vi "Get Output DMA Refs.vi"(8 "error in (no error)":errorcluster, 10 "Item GUID":string, 11 "Section Ref in":T1 format="%.0x") -> (0 "error out":errorcluster, 1 "Refs":T2(array[cluster]) {"VS Refs" format="%.0x"}, 2 "DMA":T3[](array[typedef]) {"Data Type" format="%.0x"; "DMA.Settings"."DMA Host Buffer" items=["1 Second"=1, "2 Seconds"=2, "5 Seconds"=5, "10 Seconds"=10]; "DMA.Settings"."dt" format="%#_p"; "DMA.Settings"."Update Rate" items=["1 Hz"=1, "2 Hz"=2, "5 Hz"=5, "10 Hz"=10]}, 3 "Section Ref out":T1 format="%.0x")   [LabVIEW 2020, in "FPGA Addon System Explorer.lvlib"]
uses:
  FPGA Addon System Explorer.lvlib
  <vilib>/NI VeriStand/Custom Device API/Custom Device Item Ref.ctl
  Addon Shared/Types/Compiled.DMASettings.ctl
  Addon Shared/Types/FPGA Addon Data Type.ctl
  Addon Shared/Types/DMA Settings.ctl
  Addon Shared/Types/Delacing Scheme.ctl
  Addon Shared/Types/DMA Acquisition Mode.ctl
  <vilib>/NI VeriStand/Custom Device API/Waveform Data Reference.ctl
  Addon Shared/Types/FG Action.ctl
  Addon Shared/SubVIs/Constants.vi
  <vilib>/NI VeriStand/Custom Device Tools/Custom Device Utility Library/NI VeriStand - Search for Item by GUID.vi
  <vilib>/NI/NI VeriStand Advanced SysDef API/SysDef API/SysDef.Property.Get.vi
  <vilib>/NI/NI VeriStand Advanced SysDef API/_SubVIs/SysDef.Property.Get.Variant.vi
  <vilib>/NI/NI VeriStand Advanced SysDef API/SysDef API/SysDef.Property.Set.vi
  <vilib>/NI/NI VeriStand Advanced SysDef API/_SubVIs/SysDef.Property.Set.Variant.vi
  <vilib>/NI VeriStand/Custom Device API/Get Item Property (String).vi
  <vilib>/NI VeriStand/Custom Device API/Get Item Property (U32).vi
  <vilib>/NI VeriStand/Custom Device API/Get Item Property (Double).vi
  <vilib>/NI VeriStand/Custom Device API/NI VeriStand - Set Item Property.vi
  <vilib>/NI VeriStand/Custom Device API/Set Item Property (U32).vi
  <vilib>/NI VeriStand/Custom Device API/Set Item Property (Double).vi
  <vilib>/NI VeriStand/Custom Device Tools/Custom Device Utility Library/NI VeriStand - Search for All Items by GUID.vi
  <vilib>/NI VeriStand/Custom Device API/Get Item Property (Dependent Node Pointer).vi
  Addon Shared/FPGA Addon Shared.lvlib
  <vilib>/NI VeriStand/Custom Device API/Custom Device API.lvlib
  <vilib>/NI VeriStand/Custom Device Tools/Custom Device Utility Library/Custom Device Utility Library.lvlib
  <vilib>/NI VeriStand/Custom Device Tools/Custom Device Utility Library/NI VeriStand - Search for Item by Name.vi
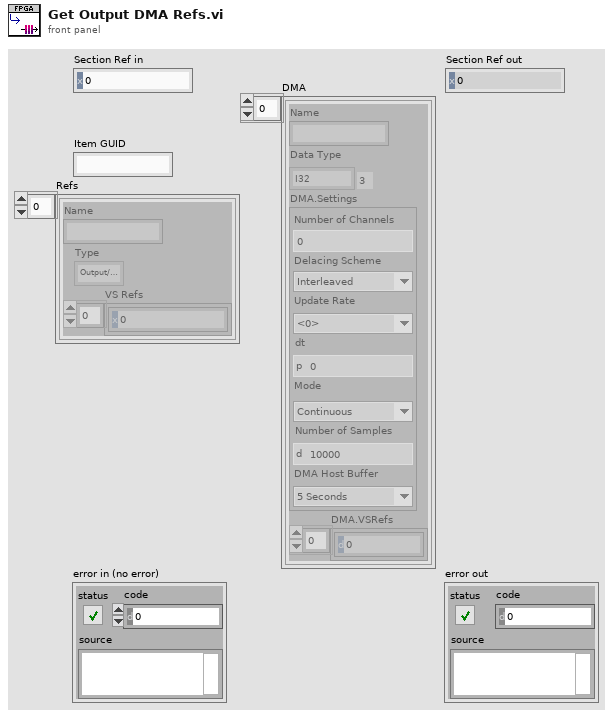
[diagram p1: front panel]
types:
  T1 = typedef "Custom Device API.lvlib/Custom Device Item Ref.ctl" = u64
  T2 = cluster{"Name":string, "Type":enum16{"Output/Write", "Input/Read", "Input/ReadWrite"}, "VS Refs":T1[]}[]
  T3 = typedef "FPGA Addon Shared.lvlib/Compiled.DMASettings.ctl" = cluster{"Name":string, "Data Type":T4, "DMA.Settings":T5, "DMA.VSRefs":T8[]}
  T4 = typedef "FPGA Addon Shared.lvlib/FPGA Addon Data Type.ctl" = enum8{"<Null>", "I8", "I16", "I32", "I64", "U8", "U16", "U32", "U64", "SGL", "Boolean", "Analog PWM In Settings", "Analog PWM In", "Digital PWM In Settings", "Digital PWM In", "Digital PWM Out", "Sine Out", "FXP", "FXP+/-24.5", "FXP+/-16.5", "FXP+/-32.8", "FXP+/-64.32", "FXP+/-16.7", "FXP+/-20.5", "FXP+/-27.5", "FXP+/-32.16", "FXP+16.3", "FXP+18.3", "Digital Static In", "Digital Static Out", "Digital Static In Settings", "Digital WSS Out", "Quad Encoder Settings", "Quad Encoder In", "Group"}
  T5 = typedef "FPGA Addon Shared.lvlib/DMA Settings.ctl" = cluster{"Number of Channels":u8, "Delacing Scheme":T6, "Update Rate":u32, "dt":dbl, "Mode":T7, "Number of Samples":u32, "DMA Host Buffer":u32}
  T6 = typedef "FPGA Addon Shared.lvlib/Delacing Scheme.ctl" = enum8{"Interleaved", "Bitpacked"}
  T7 = typedef "FPGA Addon Shared.lvlib/DMA Acquisition Mode.ctl" = enum8{"Continuous", "Triggered Finite"}
  T8 = typedef "Custom Device API.lvlib/Waveform Data Reference.ctl" = i32
  T9 = typedef "FPGA Addon Shared.lvlib/FG Action.ctl" = enum8{"GET", "SET"}
  T10 = typedef "FPGA Addon Shared.lvlib/DMA Information.ctl" = cluster{"Name":string, "Data Type":T4}
  T11 = cluster{"Name":string, "Type":enum16{"Output/Write", "Input/Read", "Input/ReadWrite"}, "VS Refs":T1[]}
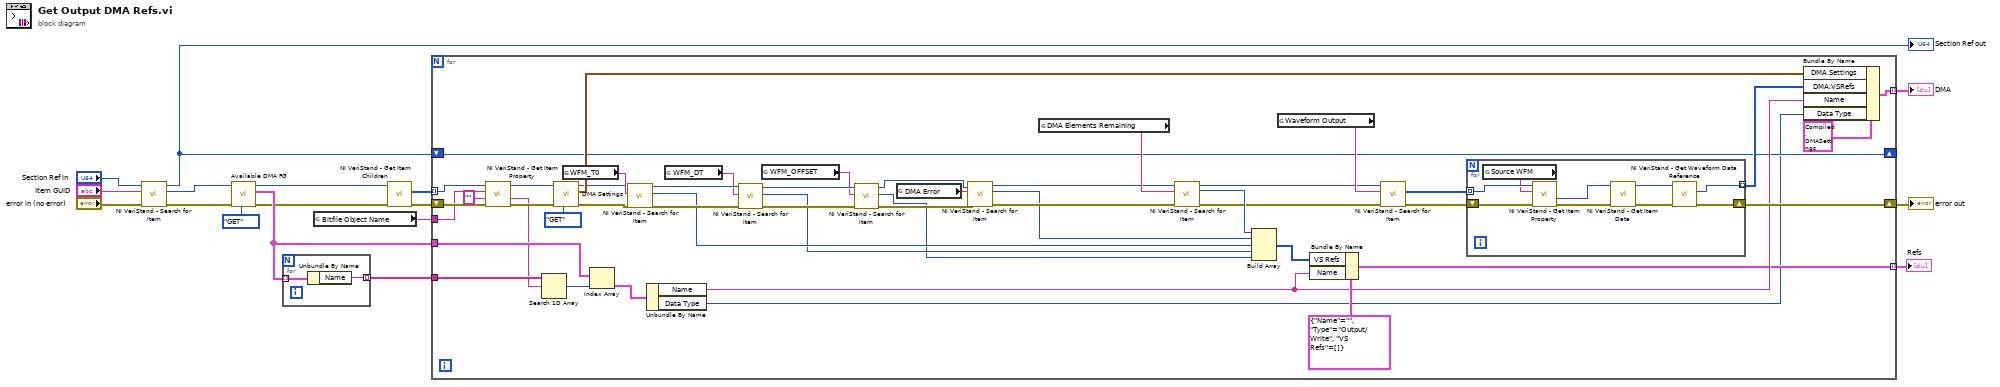
[diagram p0: block diagram]
diagram:
  n1 = call-poly <vilib>:"NI VeriStand - Search for Item.vi"("error in"="error in (no error)", "Item GUID"="Item GUID", "Section Ref in"="Section Ref in") -> ("error out"=w14:errorcluster, "Item Ref"=w16:T1, "Section Ref out"=w3:T1)  [unwired: 5 in, 1 out]
  "Section Ref out" <- w3
  n2 = call "Available DMA FG.vi"("Action"=FG_Action."GET", "error in (no error)"=w14, "Item Ref"=w16) -> ("error out"=w10:errorcluster, "Available DMA"=w11:T10[], "Item Ref out"=w12:T1)  [unwired: 6 in]
  n3 = for {
    tunnel: w11 -> [w19] mode=indexing
    tunnel: [w18] -> w9 mode=indexing
    n4 = Unbundle By Name(w19) -> ("Name"=w18:string)
  }
  n5 = global read "Constants.vi" "Bitfile Object Name"() -> (w8:string)
  n6 = call <vilib>:"NI VeriStand - Get Item Children.vi"("error in (no error)"=w10, "Item Ref in"=w12) -> ("error out"=w6:errorcluster, "Child Refs"=w7:T1[])  [unwired: 6 in, 2 out]
  n7 = for {
    shift-right: [w42] -> w4
    shift-left: w6 -> [w67]
    tunnel: w7 -> [w66] mode=indexing
    tunnel: w8 -> [w65]
    tunnel: w9 -> [w63]
    tunnel: w11 -> [w62]
    tunnel: [w57] -> w2 mode=indexing
    shift-right: [w35] -> _
    shift-left: w3 -> [w35]
    tunnel: [w37] -> w1 mode=indexing
    n8 = call-poly <vilib>:"NI VeriStand - Get Item Property.vi"("error in (no error)"=w67, "Default Value"="", "Property Name"=w65, "Item Ref in"=w66) -> ("error out"=w56:errorcluster, "Value"=w52:string, "Item Ref out"=w55:T1)  [unwired: 4 in, 1 out]
    n9 = Search 1D Array(1D array=w63, element=w52) -> (index of element=w61:i32)  [unwired: 1 in]
    n10 = call "DMA Settings.vi"("Action"=FG_Action."GET", "error in (no error)"=w56, "Item Ref"=w55) -> ("error out"=w23:errorcluster, "DMA Settings"=w44:T5, "Item Ref out"=w24:T1)  [unwired: 6 in]
    n11 = global read "Constants.vi" "WFM_T0"() -> (w29:string)
    n12 = Index Array(array=w62, index=w61) -> (element=w59:T10)
    n13 = call-poly <vilib>:"NI VeriStand - Search for Item.vi"("error in"=w23, "Item Name"=w29, "Section Ref in"=w24) -> ("error out"=w32:errorcluster, "Item Ref"=w22:T1, "Section Ref out"=w33:T1)  [unwired: 5 in, 1 out]
    n14 = Unbundle By Name(w59) -> ("Name"=w38:string, "Data Type"=w34:T4)
    n15 = global read "Constants.vi" "WFM_DT"() -> (w28:string)
    n16 = call-poly <vilib>:"NI VeriStand - Search for Item.vi"("error in"=w32, "Item Name"=w28, "Section Ref in"=w33) -> ("error out"=w30:errorcluster, "Item Ref"=w21:T1, "Section Ref out"=w31:T1)  [unwired: 5 in, 1 out]
    n17 = global read "Constants.vi" "WFM_OFFSET"() -> (w27:string)
    n18 = call-poly <vilib>:"NI VeriStand - Search for Item.vi"("error in"=w30, "Item Name"=w27, "Section Ref in"=w31) -> ("error out"=w25:errorcluster, "Item Ref"=w20:T1, "Section Ref out"=w26:T1)  [unwired: 5 in, 1 out]
    n19 = global read "Constants.vi" "DMA Error"() -> (w51:string)
    n20 = call-poly <vilib>:"NI VeriStand - Search for Item.vi"("error in"=w25, "Item GUID"=w51, "Section Ref in"=w26) -> ("error out"=w49:errorcluster, "Item Ref"=w47:T1, "Section Ref out"=w48:T1)  [unwired: 5 in, 1 out]
    n21 = global read "Constants.vi" "DMA Elements Remaining"() -> (w50:string)
    n22 = call-poly <vilib>:"NI VeriStand - Search for Item.vi"("error in"=w49, "Item GUID"=w50, "Section Ref in"=w48) -> ("error out"=w36:errorcluster, "Item Ref"=w46:T1, "Section Ref out"=w45:T1)  [unwired: 5 in, 1 out]
    n23 = Build Array(w46, w47, w22, w21, w20) -> (w39:T1[])
    n24 = global read "Constants.vi" "Waveform Output"() -> (w53:string)
    n25 = Bundle By Name(cluster=T11 {"Name"="", "Type"=enum."Output/Write", "VS Refs"=[]} ("Group"), "VS Refs"=w39, "Name"=w38) -> (w37:T11)
    n26 = call-poly <vilib>:"NI VeriStand - Search for Item.vi"("error in"=w36, "Item GUID"=w53, "Section Ref in"=w45) -> ("error out"=w54:errorcluster, "Item Refs"=w43:T1[])  [unwired: 5 in, 2 out]
    n27 = for {
      shift-right: [w68] -> w42
      shift-left: w54 -> [w76]
      tunnel: [w69] -> w41 mode=indexing
      tunnel: w43 -> [w75] mode=indexing
      n28 = global read "Constants.vi" "Source WFM"() -> (w74:string)
      n29 = call-poly <vilib>:"NI VeriStand - Get Item Property.vi"("error in (no error)"=w76, "Property Name"=w74, "Item Ref in"=w75) -> ("error out"=w73:errorcluster, "Dependent Node Ref"=w71:T1)  [unwired: 5 in, 2 out]
      n30 = call <vilib>:"NI VeriStand - Get Item Data.vi"("error in (no error)"=w73, "Item Ref in"=w71) -> ("error out"=w72:errorcluster, "Item Ref out"=w70:T1)  [unwired: 8 out]
      n31 = call <vilib>:"NI VeriStand - Get Waveform Data Reference.vi"("error in (no error)"=w72, "Waveform Ref in"=w70) -> ("error out"=w68:errorcluster, "Waveform Data Reference"=w69:T8)  [unwired: 7 in, 1 out]
    }
    n32 = Bundle By Name(cluster=T3 {"Name"="", "Data Type"=enum."I32", "DMA.Settings"={"Number of Channels"=0, "Delacing Scheme"=enum."Interleaved", "Update Rate"=0, "dt"=0.0, "Mode"=enum."Continuous", "Number of Samples"=10000, "DMA Host Buffer"=5}, "DMA.VSRefs"=[]}, "DMA.Settings"=w44, "DMA.VSRefs"=w41, "Name"=w38, "Data Type"=w34) -> (w57:T3)
  }
  "error out" <- w4
  "DMA" <- w2
  "Refs" <- w1
